vi "Action_1.vi"(1 "Time Since Latch":u32, 2 "Instruction String":string) -> (0 "Advance Trigger":bool)   [LabVIEW 2018]
uses:
  Global_Commands.vi
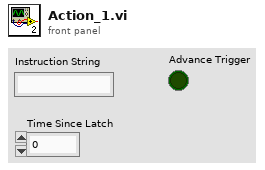
[diagram p1: front panel]
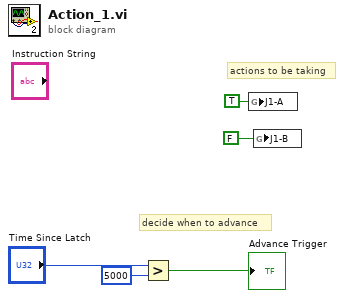
[diagram p0: block diagram]
diagram:
  # "actions to be taking"
  # "decide when to advance"
  n1 = Greater?(x="Time Since Latch", y=u32 5000) -> (0:→"Advance Trigger":bool)
  n2 = global write "Global_Commands.vi" "J1-A"(TRUE ("J1-A")) -> ()
  n3 = global write "Global_Commands.vi" "J1-B"(FALSE) -> ()
